vi "Create Ansiotropic Filter 32f.vi"(8 "Error In":errorcluster, 9 "Dimensions":T1={"Depth"=1, "Height"=1, "Width"=1} {"Width" min=1; "Height" min=1; "Depth" min=1}, 10 "Ansiotropic Filter Parameters":T9={"Time Step"=0.0, "Total Time"=0.5, "Std. Deviation"=0.0, "Gaussian Filter X Size"=1, "Gaussian Filter Y Size"=1, "Gaussian Filter Z Size"=1} {"Gaussian Filter Z Size" min=1 max=99 step=2; "Gaussian Filter Y Size" min=1 max=99 step=2; "Gaussian Filter X Size" min=1 max=99 step=2}, 11 "Device In":T3) -> (0 "Error Out":errorcluster, 3 "Anisotropic Filter Object":T2={"Device In"=0, "Convolution Object"={"Device In"=0, "Program Handle"=0, "Kernel Memory Object"={"Device ID"=0, "Memeroy ID"=0, "Dimension"={"Depth"=0, "Height"=0, "Width"=0}, "Memory Type"=enum."32f"}, "Convolved Memory Object"={"Device ID"=0, "Memeroy ID"=0, "Dimension"={"Depth"=0, "Height"=0, "Width"=0}, "Memory Type"=enum."32f"}}, "Imag Kernel"=[], "Real Kernel"=[], "Convolved Buffer"={"Device ID"=0, "Memeroy ID"=0, "Dimension"={"Depth"=0, "Height"=0, "Width"=0}, "Memory Type"=enum."32f"}, "Program Handle"=0, "Ansiotropic Filter Parameters"={"Time Step"=0.0, "Total Time"=0.5, "Std. Deviation"=0.0, "Gaussian Filter X Size"=1, "Gaussian Filter Y Size"=1, "Gaussian Filter Z Size"=1}, "Raw Data"={"Device ID"=0, "Memeroy ID"=0, "Dimension"={"Depth"=0, "Height"=0, "Width"=0}, "Memory Type"=enum."32f"}, "Buffer 3"={"Device ID"=0, "Memeroy ID"=0, "Dimension"={"Depth"=0, "Height"=0, "Width"=0}, "Memory Type"=enum."32f"}, "Dimensions"={"Depth"=1, "Height"=1, "Width"=1}} {"Dimensions"."Width" min=1; "Dimensions"."Height" min=1; "Dimensions"."Depth" min=1; "Buffer 3"."Dimension"."Width" min=1; "Buffer 3"."Dimension"."Height" min=1; "Buffer 3"."Dimension"."Depth" min=1; "Raw Data"."Dimension"."Width" min=1; "Raw Data"."Dimension"."Height" min=1; "Raw Data"."Dimension"."Depth" min=1; "Ansiotropic Filter Parameters"."Gaussian Filter Z Size" min=1 max=99 step=2; "Ansiotropic Filter Parameters"."Gaussian Filter Y Size" min=1 max=99 step=2; "Ansiotropic Filter Parameters"."Gaussian Filter X Size" min=1 max=99 step=2; "Convolved Buffer"."Dimension"."Width" min=1; "Convolved Buffer"."Dimension"."Height" min=1; "Convolved Buffer"."Dimension"."Depth" min=1; "Convolution Object"."Convolved Memory Object"."Dimension"."Width" min=1; "Convolution Object"."Convolved Memory Object"."Dimension"."Height" min=1; "Convolution Object"."Convolved Memory Object"."Dimension"."Depth" min=1; "Convolution Object"."Kernel Memory Object"."Dimension"."Width" min=1; "Convolution Object"."Kernel Memory Object"."Dimension"."Height" min=1; "Convolution Object"."Kernel Memory Object"."Dimension"."Depth" min=1})   [LabVIEW 2012, in "OpenCLV x64.lvlib"]
doc: "Creates an Anisotropic Filter Object that contains the program and all memory objects needed for the filter."
uses:
  OpenCLV x64.lvlib
  Controls/Anisotropic Filter Parameters.ctl
  Controls/Device ID.ctl
  Controls/Anisotropic Filter Object.ctl
  Controls/Convolution Object.ctl
  Controls/Program Handle.ctl
  Controls/Memory Object.ctl
  Controls/Memory ID.ctl
  User Controls/Array Dimensions.ctl
  Controls/Memory Type.ctl
  Allocate Memory/AllocateMemory_32f.vi
  Convolution/Create Convolution 32f.vi
panel:
  out "Imag Kernel":sgl[][][](array[numeric])
  out "Real Kernel":sgl[][][](array[numeric])
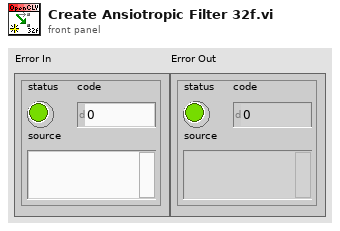
[diagram p1: front panel]
types:
  T1 = typedef "Array Dimensions.ctl" = cluster{"Depth":u64, "Height":u64, "Width":u64}
  T2 = typedef "OpenCLV x64.lvlib/Anisotropic Filter Object.ctl" = cluster{"Device In":T3, "Convolution Object":T4, "Imag Kernel":sgl[][][], "Real Kernel":sgl[][][], "Convolved Buffer":T6, "Program Handle":T5, "Ansiotropic Filter Parameters":T9, "Raw Data":T6, "Buffer 3":T6, "Dimensions":T1}
  T3 = typedef "OpenCLV x64.lvlib/Device ID.ctl" = u64
  T4 = typedef "OpenCLV x64.lvlib/Convolution Object.ctl" = cluster{"Device In":T3, "Program Handle":T5, "Kernel Memory Object":T6, "Convolved Memory Object":T6}
  T5 = typedef "OpenCLV x64.lvlib/Program Handle.ctl" = u64
  T6 = typedef "OpenCLV x64.lvlib/Memory Object.ctl" = cluster{"Device ID":T3, "Memeroy ID":T7, "Dimension":T1, "Memory Type":T8}
  T7 = typedef "OpenCLV x64.lvlib/Memory ID.ctl" = u64
  T8 = typedef "OpenCLV x64.lvlib/Memory Type.ctl" = enum16{"32f", "u8", "i8", "u16", "i16", "u32", "i32", "64f"}
  T9 = typedef "OpenCLV x64.lvlib/Anisotropic Filter Parameters.ctl" = cluster{"Time Step":sgl, "Total Time":sgl, "Std. Deviation":sgl, "Gaussian Filter X Size":u32, "Gaussian Filter Y Size":u32, "Gaussian Filter Z Size":u32}
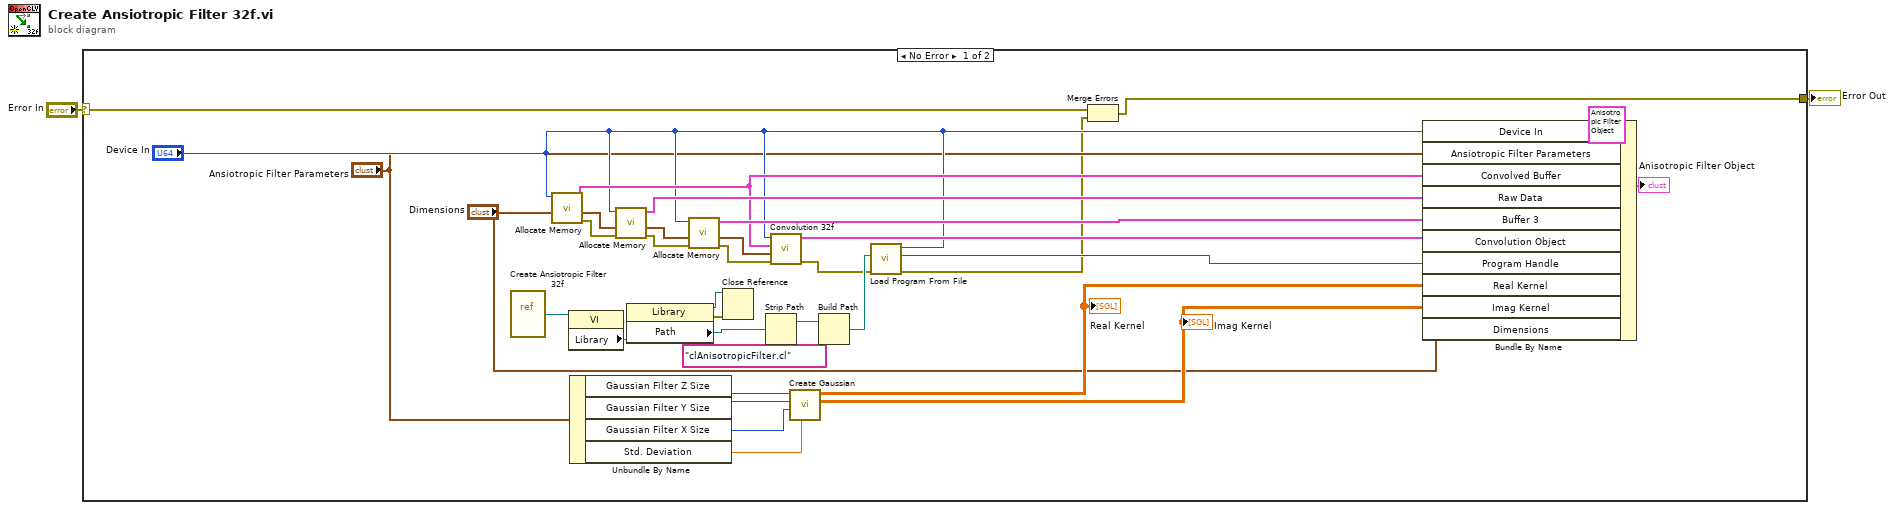
[diagram p0: block diagram]
diagram:
  n1 = case shown="No Error" "Error In" {
    selector: "Error In" -> [w5 w37]
    tunnel: [w4 w37] -> w1
    frame No Error {
      n2 = vi-ref "Create Ansiotropic Filter 32f.vi"() -> (w30:refnum<vi>)
      n3 = call-poly "Allocate Memory.vi"("Dimension"="Dimensions", "Device In"="Device In") -> ("Error Out"=w23:errorcluster, "Dimension Out"=w22:T1, "Memory Object"=w18:T6)  [unwired: 7 in]
      n4 = property class="VI"(reference=w30) -> ("Library"=w32:refnum<vi>)  [unwired: 1 in, 2 out]
      n5 = Unbundle By Name("Ansiotropic Filter Parameters") -> ("Gaussian Filter Z Size"=w12:u32, "Gaussian Filter Y Size"=w10:u32, "Gaussian Filter X Size"=w9:u32, "Std. Deviation"=w11:sgl)
      n6 = call-poly "Allocate Memory.vi"("Error In"=w23, "Dimension"=w22, "Device In"="Device In") -> ("Error Out"=w27:errorcluster, "Dimension Out"=w28:T1, "Memory Object"=w21:T6)  [unwired: 6 in]
      n7 = property class="Library"(reference=w32) -> (reference out=w7:refnum<vi>, error out=w8:errorcluster, "Path"=w31:path)  [unwired: 1 in]
      n8 = call-poly "Allocate Memory.vi"("Error In"=w27, "Dimension"=w28, "Device In"="Device In") -> ("Error Out"=w16:errorcluster, "Dimension Out"=w3:T1, "Memory Object"=w20:T6)  [unwired: 6 in]
      n9 = Close Reference(reference=w7, error in (no error)=w8) -> ()  [unwired: 1 out]
      n10 = Strip Path(path=w31) -> (stripped path=w34:path)  [unwired: 1 out]
      n11 = call-poly "Convolution 32f.vi"("Error In"=w16, "Convolution Dimensions"=w3, "Memory Object"=w18, "Device In"="Device In") -> ("Error Out"=w15:errorcluster, "Convolution Object"=w19:T4)  [unwired: 6 in]
      n12 = call "Create Gaussian.vi"("Std. Deviation"=w11, "Gaussian Filter X Size"=w9, "Gaussian Filter Y Size"=w10, "Gaussian Filter Z Size"=w12) -> ("Array 2"=w29:sgl[][][], "Array"=w26:sgl[][][])  [unwired: 6 in]
      "Real Kernel" <- w26
      "Imag Kernel" <- w29
      n13 = Build Path(base path=w34, name or relative path="clAnisotropicFilter.cl") -> (appended path=w25:path)
      n14 = call "Load Program From File.vi"("Error In"=w15, "Program Path"=w25, "Device In"="Device In") -> ("Error Out"=w6:errorcluster, "Program Handle"=w24:T5)  [unwired: 6 in, 1 out]
      n15 = Merge Errors(w5, w6) -> (w4:errorcluster)
      n16 = Bundle By Name(cluster=T2 {"Device In"=0, "Convolution Object"={"Device In"=0, "Program Handle"=0, "Kernel Memory Object"={"Device ID"=0, "Memeroy ID"=0, "Dimension"={"Depth"=0, "Height"=0, "Width"=0}, "Memory Type"=enum."32f"}, "Convolved Memory Object"={"Device ID"=0, "Memeroy ID"=0, "Dimension"={"Depth"=0, "Height"=0, "Width"=0}, "Memory Type"=enum."32f"}}, "Imag Kernel"=[], "Real Kernel"=[], "Convolved Buffer"={"Device ID"=0, "Memeroy ID"=0, "Dimension"={"Depth"=0, "Height"=0, "Width"=0}, "Memory Type"=enum."32f"}, "Program Handle"=0, "Ansiotropic Filter Parameters"={"Time Step"=0.0, "Total Time"=0.0, "Std. Deviation"=0.0, "Gaussian Filter X Size"=0, "Gaussian Filter Y Size"=0, "Gaussian Filter Z Size"=0}, "Raw Data"={"Device ID"=0, "Memeroy ID"=0, "Dimension"={"Depth"=0, "Height"=0, "Width"=0}, "Memory Type"=enum."32f"}, "Buffer 3"={"Device ID"=0, "Memeroy ID"=0, "Dimension"={"Depth"=0, "Height"=0, "Width"=0}, "Memory Type"=enum."32f"}, "Dimensions"={"Depth"=0, "Height"=0, "Width"=0}} ("Anisotropic Filter Object"), "Device In"="Device In", "Ansiotropic Filter Parameters"="Ansiotropic Filter Parameters", "Convolved Buffer"=w18, "Raw Data"=w21, "Buffer 3"=w20, "Convolution Object"=w19, "Program Handle"=w24, "Real Kernel"=w26, "Imag Kernel"=w29, "Dimensions"="Dimensions") -> (→"Anisotropic Filter Object":T2)
    }
    frame Error {
    }
  }
  "Error Out" <- w1
